vi "Configure Ethernet Autostart.vi"(0 "VISA resource name":refnum<visa-resource-name>, 5 "Autostart Enabled":bool, 11 "error in (no error)":errorcluster) -> (4 "VISA resource name out":refnum<visa-resource-name>, 15 "error out":errorcluster)   [LabVIEW 2016, in "APT 300XAC Series.lvlib"]
doc: "Sets the Autostart Mode Of the APT 300XAC Series Power Source instrument"
uses:
  APT 300XAC Series.lvlib
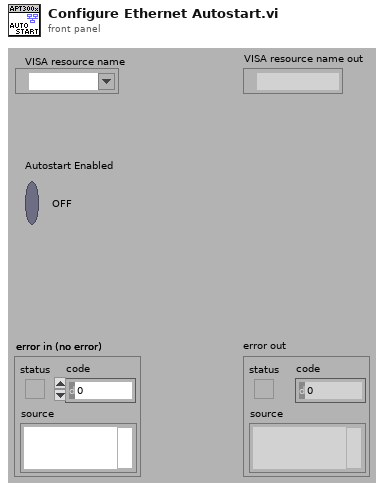
[diagram p1: front panel]
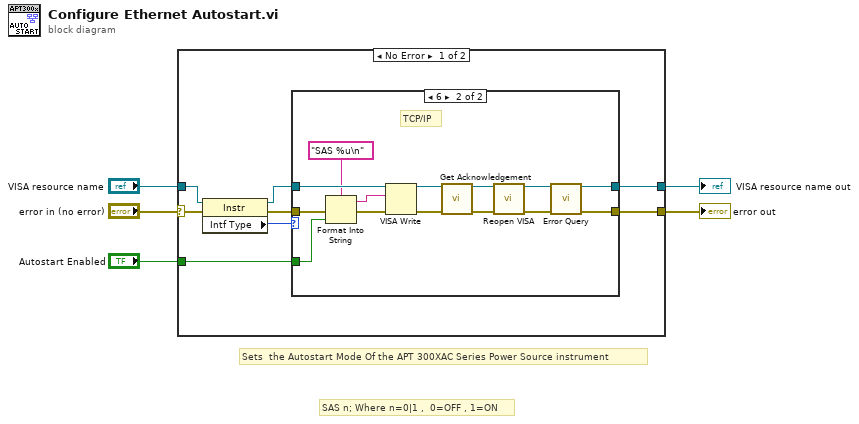
[diagram p0: block diagram]
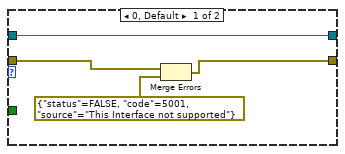
[diagram p2: hidden frame]
diagram:
  # "SAS n; Where n=0|1 ,  0=OFF , 1=ON"
  # "Sets  the Autostart Mode Of the APT 300XAC Series Power Source instrument"
  n1 = case shown="No Error" "error in (no error)" {
    selector: "error in (no error)" -> [w11 w33]
    tunnel: "VISA resource name" -> [w8 w32]
    tunnel: [w13 w32] -> w1
    tunnel: [w12 w33] -> w2
    tunnel: "Autostart Enabled" -> [w10 _]
    frame No Error {
      n2 = property class="Instr"(reference=w8, error in=w11) -> (reference out=w7:refnum<visa-resource-name>, error out=w9:errorcluster, "Intf Type"=w6:u16)
      n3 = case shown="6" w6 {
        tunnel: w7 -> [w17 w31]
        tunnel: [w17 w30] -> w13
        tunnel: [w14 w28] -> w12
        tunnel: w9 -> [w15 w18]
        tunnel: w10 -> [_ w24]
        frame 0, Default {
          n4 = Merge Errors(w15, errorcluster {"status"=FALSE, "code"=5001, "source"="This Interface not supported"} ("error in 2 (no error)")) -> (w14:errorcluster)
        }
        frame 6 {
          # "TCP/IP"
          n5 = Format Into String(format string="SAS %u\n" ("Command to Send"), error in=w18, w24) -> (resulting string=w27:string, error out=w26:errorcluster)  [unwired: 1 in]
          n6 = VISA Write(VISA resource name=w31, write buffer=w27, error in (no error)=w26) -> (VISA resource name out=w22:refnum<visa-resource-name>, error out=w29:errorcluster)  [unwired: 1 out]
          n7 = call "Get Acknowledgement.vi"("VISA resource name"=w22, "error in (no error)"=w29) -> ("VISA resource name out"=w20:refnum<visa-resource-name>, "error out"=w23:errorcluster)  [unwired: 12 in]
          n8 = call "Reopen VISA.vi"("VISA resource name"=w20, "error in (no error)"=w23) -> ("VISA resource name out"=w19:refnum<visa-resource-name>, "error out"=w21:errorcluster)  [unwired: 12 in]
          n9 = call "Error Query.vi"("VISA resource name"=w19, "error in (no error)"=w21) -> ("VISA resource name out"=w30:refnum<visa-resource-name>, "error out"=w28:errorcluster)  [unwired: 10 in, 2 out]
        }
      }
    }
    frame Error {
    }
  }
  "error out" <- w2
  "VISA resource name out" <- w1
